vi "Tokenize Record String.vi"(11 "Record String":string) -> (1 "Payload Binary":string, 2 "Datatype":string, 3 "Record Type":string)   [LabVIEW 2019, in "ParseGDSII.lvclass"]
uses:
  ParseGDSII.lvclass
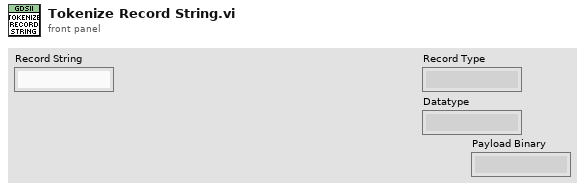
[diagram p1: front panel]
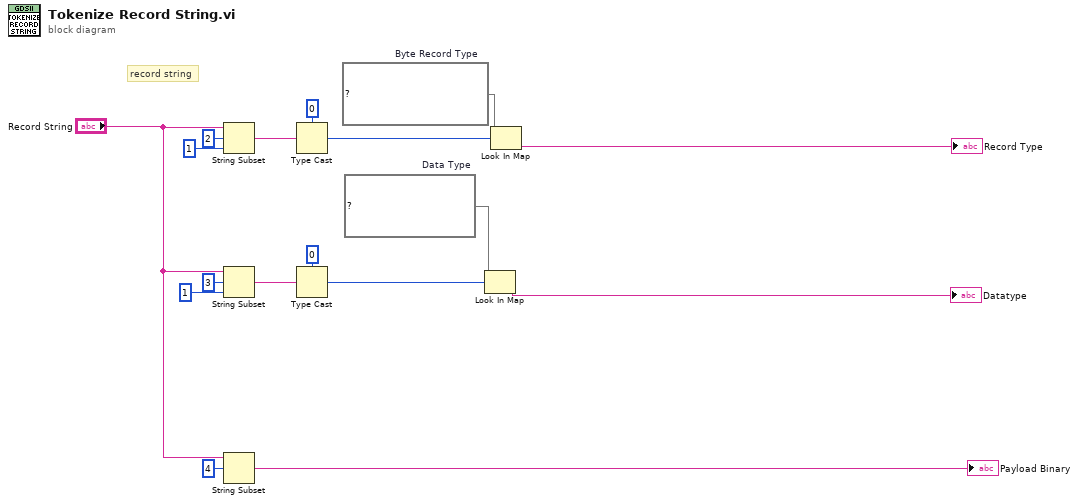
[diagram p0: block diagram]
diagram:
  w2 = map{i8, string} {0="No Data", 1="Bit Array", 2="Word", 3="Long", 5="Real", 6="String"}  # Data Type
  w5 = map{i32, string} {0="HEADER", 1="BGNLIB", 2="LIBNAME", 3="UNITS", 4="ENDLIB", 5="BGNSTR", 6="STRNAME", 7="ENDSTR", 8="BOUNDARY", 9="PATH", 10="SREF", 11="AREF", 12="TEXT", 13="LAYER", 14="DATATYPE", 15="WIDTH", 16="XY", 17="ENDEL", 18="SNAME", 19="COLROW", 21="NODE", 22="TEXTTYPE", 23="PRESENTATION", 25="STRING", 26="STRANS", 27="MAG", 28="ANGLE", 31="REFLIBS", 32="FONTS", 33="PATHTYPE", 34="GENERATIONS", 35="ATTRTABLE", 38="ELFLAGS", 42="NODETYPE", 43="PROPATTR", 44="PROPVALUE", 45="BOX", 46="BOXTYPE", 47="PLEX", 50="TAPENUM", 51="TAPECODE", 54="FORMAT", 55="MASK", 56="ENDMASKS"}  # Byte Record Type
  # "record string"
  n1 = String Subset(string="Record String", offset (0)=2, length (rest)=1 ("length (rest)")) -> (substring=w13:string)
  n2 = String Subset(string="Record String", offset (0)=3, length (rest)=1 ("length (rest)")) -> (substring=w11:string)
  n3 = String Subset(string="Record String", offset (0)=4) -> (substring=→"Payload Binary":string)  [unwired: 1 in]
  n4 = Type Cast(type=i8 0, x=w13) -> (*(type *) &x=w8:i8)
  n5 = Type Cast(type=i8 0, x=w11) -> (*(type *) &x=w7:i8)
  n6 = Look In Map(map=w2, key=w7) -> (value=→"Datatype":string)  [unwired: 1 in, 1 out]
  n7 = Look In Map(map=w5, key=w8) -> (value=→"Record Type":string)  [unwired: 1 in, 1 out]
